vi "test.vi"() -> ()   [LabVIEW 2017]
panel:
  out "error out 2":errorcluster
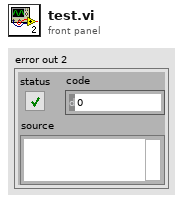
[diagram p1: front panel]
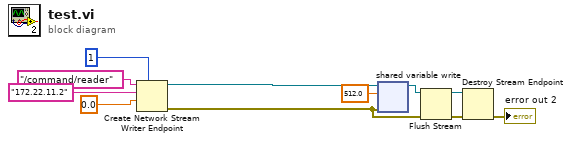
[diagram p0: block diagram]
diagram:
  n1 = Create Network Stream Writer Endpoint(7:1 ("writer buffer size"), 9:0.0, 10:"172.22.11.2" ("reader url"), 11:"/command/reader" ("writer name")) -> (0:w3:errorcluster, 3:w7:refnum<k21>)  [unwired: 3 in]
  n2 = shared-variable-write(w7, w3, 512.0 ("data in")) -> (w2:refnum<k21>)  [unwired: 1 in, 2 out]
  n3 = Flush Stream(8:w3, 11:w2) -> (0:w6:errorcluster, 3:w5:refnum<k21>)  [unwired: 2 in, 1 out]
  n4 = Destroy Stream Endpoint(8:w6, 11:w5) -> (0:→"error out 2":errorcluster)
